vi "Position.vi"(8 "error in (no error)":errorcluster, 11 "Number in":refnum<class "Symbol.lvclass">) -> (0 "error out":errorcluster, 2 "Position":T1, 3 "Number out":refnum<class "Symbol.lvclass">)   [LabVIEW 2020, in "Symbol.lvclass"]
uses:
  Symbol.lvclass
  Coordinate.ctl
  Symbol.lvclass/Symbol.ctl
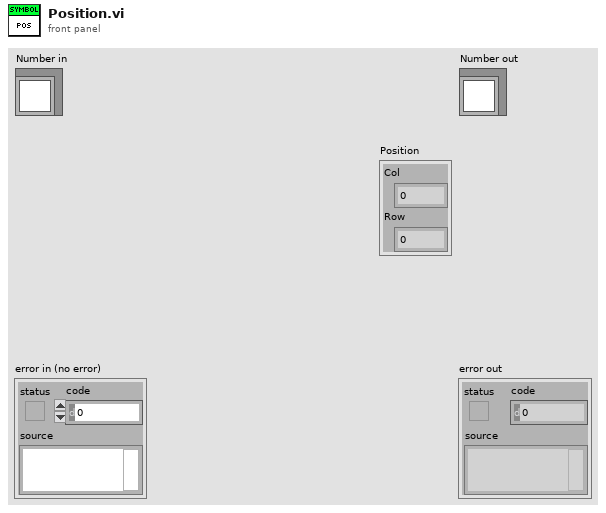
[diagram p1: front panel]
types:
  T1 = typedef "Symbol.lvclass/Coordinate.ctl" = cluster{"Col":i32, "Row":i32}
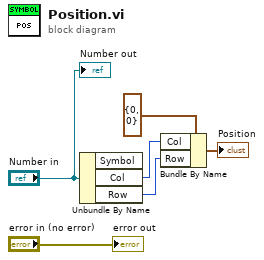
[diagram p0: block diagram]
diagram:
  n1 = Unbundle By Name("Number in") -> ("Col"=w4:i32, "Row"=w2:i32)  [unwired: 1 out]
  n2 = Bundle By Name(cluster=T1 {"Col"=0, "Row"=0} ("Position"), "Col"=w4, "Row"=w2) -> (→"Position":T1)
  "error out" <- "error in (no error)"
  "Number out" <- "Number in"
